vi "AlAs-GaAs superlattice-111203 a.vi"() -> ()   [LabVIEW 2011]
panel:
  in  "Number of \nGrowth Steps":i32=50
  out "step number":i32
  in  "Aluminum Flow":dbl=10.0
  in  "Ga Flow 1":dbl=5.49
  in  "As_Gas Flow":dbl=33.0
  in  "Manifold H2 Flow":dbl=700.0
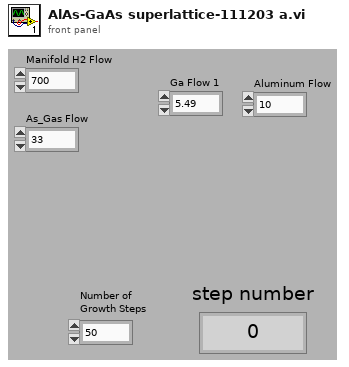
[diagram p1: front panel]
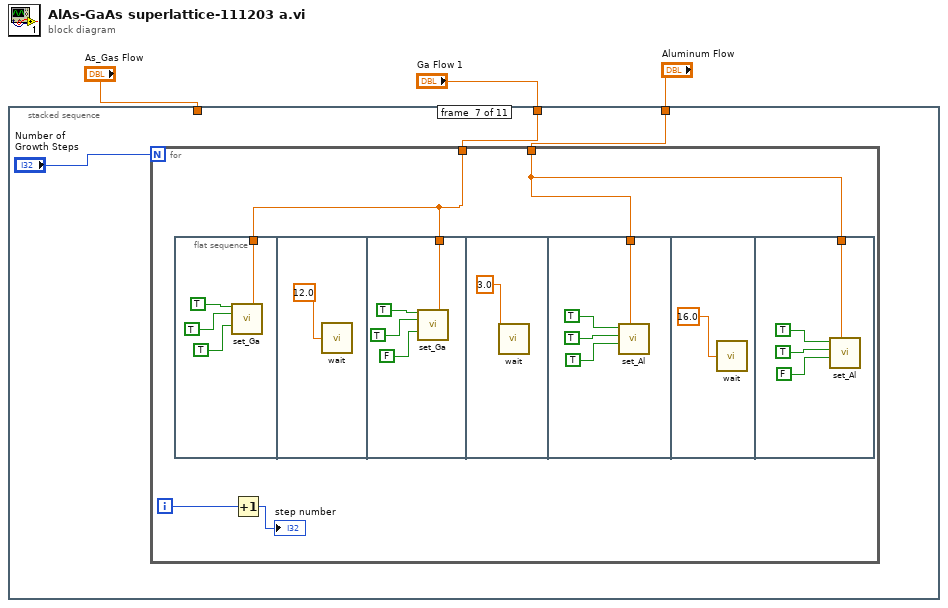
[diagram p0: block diagram]
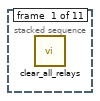
[diagram p2: hidden frame]
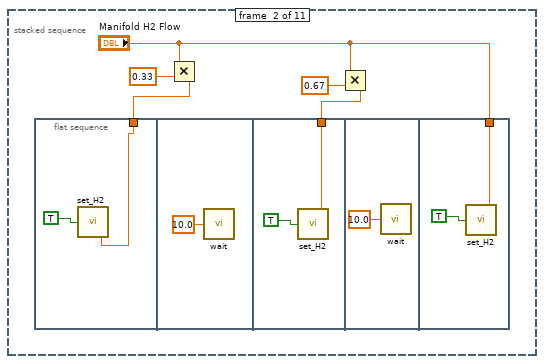
[diagram p3: hidden frame]
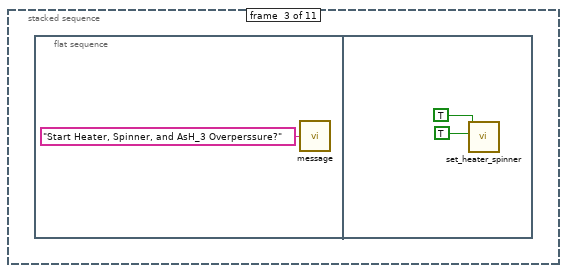
[diagram p4: hidden frame]
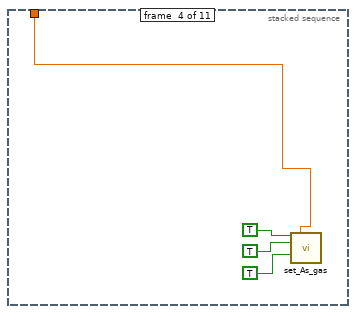
[diagram p5: hidden frame]
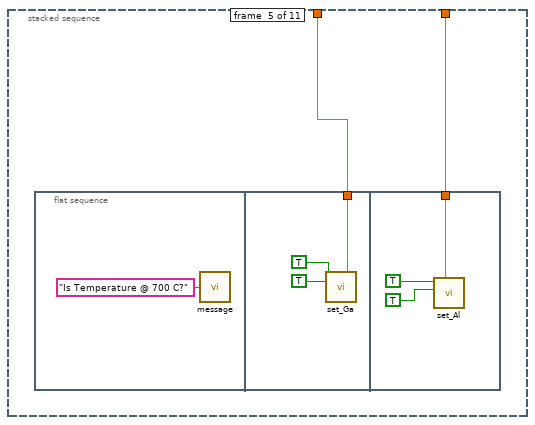
[diagram p6: hidden frame]
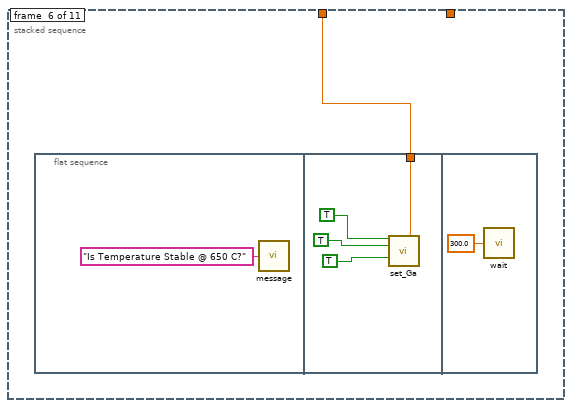
[diagram p7: hidden frame]
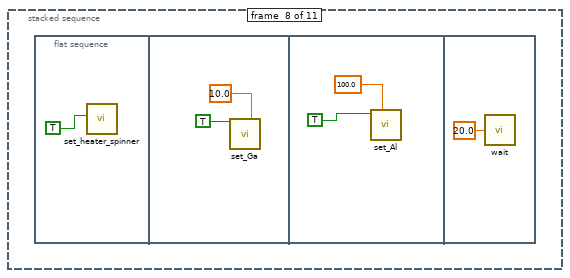
[diagram p8: hidden frame]
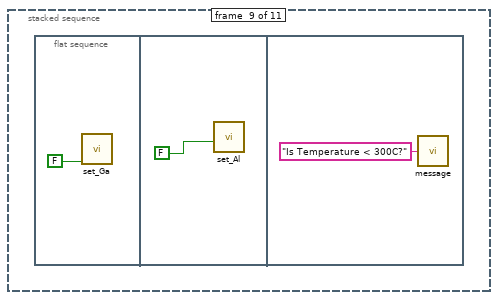
[diagram p9: hidden frame]
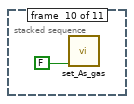
[diagram p10: hidden frame]
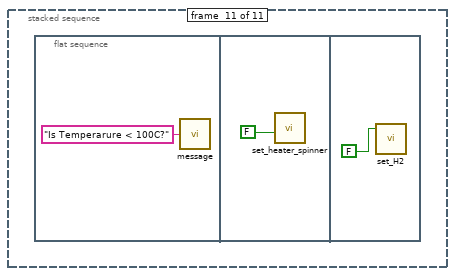
[diagram p11: hidden frame]
diagram:
  n1 = stacked-sequence {
    tunnel: "Ga Flow 1" -> [_ _ _ _ w25 w33 w41 _ _ _ _]
    tunnel: "As_Gas Flow" -> [_ _ _ w20 _ _ _ _ _ _ _]
    tunnel: "Aluminum Flow" -> [_ _ _ _ w24 _ w40 _ _ _ _]
    frame #0 {
      n2 = call "clear_all_relays.vi"() -> ()  [unwired: 2 out]
    }
    frame #1 {
      n3 = flat-sequence {
        tunnel: w8 -> [w9]
        tunnel: w6 -> [w12]
        tunnel: "Manifold H2 Flow" -> [w15]
        frame #0 {
          n4 = call "set_H2.vi"("Manifold H2 Flow"=w9, "H2 Active"=TRUE) -> ()  [unwired: 2 in, 2 out]
        }
        frame #1 {
          n5 = call "wait.vi"("Wait (s)"=10.0) -> ()
        }
        frame #2 {
          n6 = call "set_H2.vi"("Manifold H2 Flow"=w12, "H2 Active"=TRUE) -> ()  [unwired: 2 in, 2 out]
        }
        frame #3 {
          n7 = call "wait.vi"("Wait (s)"=10.0) -> ()
        }
        frame #4 {
          n8 = call "set_H2.vi"("Manifold H2 Flow"=w15, "H2 Active"=TRUE) -> ()  [unwired: 2 in, 2 out]
        }
      }
      n9 = Multiply(x="Manifold H2 Flow", y=0.33) -> (x*y=w8:dbl)
      n10 = Multiply(x="Manifold H2 Flow", y=0.67) -> (x*y=w6:dbl)
    }
    frame #2 {
      n11 = flat-sequence {
        frame #0 {
          n12 = call "message.vi"("message"="Start Heater, Spinner, and AsH_3 Overperssure?") -> ()
        }
        frame #1 {
          n13 = call "set_heater_spinner.vi"("Spinner"=TRUE, "Heater"=TRUE) -> ()  [unwired: 1 in, 7 out]
        }
      }
    }
    frame #3 {
      n14 = call "set_As_gas.vi"("As_Gas Active"=TRUE, "As_Gas Flow"=w20, "As_Gas In"=TRUE, "As_Gas Run"=TRUE) -> ()  [unwired: 2 in, 10 out]
    }
    frame #4 {
      n15 = flat-sequence {
        tunnel: w25 -> [w27]
        tunnel: w24 -> [w30]
        frame #0 {
          n16 = call "message.vi"("message"="Is Temperature @ 700 C?") -> ()
        }
        frame #1 {
          n17 = call "set_Ga.vi"("Ga Active"=TRUE, "Ga Flow 1"=w27, "Ga Bubbler"=TRUE) -> ()  [unwired: 5 in, 8 out]
        }
        frame #2 {
          n18 = call "set_Al.vi"("Aluminum Flow"=w30, "Al Bubbler"=TRUE ("Ga Bubbler"), "Al Active"=TRUE ("Ga Active")) -> ()  [unwired: 2 in, 5 out]
        }
      }
    }
    frame #5 {
      n19 = flat-sequence {
        tunnel: w33 -> [w35]
        frame #0 {
          n20 = call "message.vi"("message"="Is Temperature Stable @ 650 C?") -> ()
        }
        frame #1 {
          n21 = call "set_Ga.vi"("Ga Active"=TRUE ("P_Gas Active"), "Ga Flow 1"=w35, "Ga Bubbler"=TRUE ("P_Gas In"), "Ga Run"=TRUE ("P_Gas Run")) -> ()  [unwired: 4 in, 8 out]
        }
        frame #2 {
          n22 = call "wait.vi"("Wait (s)"=300.0) -> ()
        }
      }
    }
    frame #6 {
      n23 = for {
        N: "Number of \nGrowth Steps" -> [_]
        tunnel: w41 -> [w44]
        tunnel: w40 -> [w43]
        i -> [w45]
        n24 = flat-sequence {
          tunnel: w44 -> [w47]
          tunnel: w44 -> [w52]
          tunnel: w43 -> [w57]
          tunnel: w43 -> [w62]
          frame #0 {
            n25 = call "set_Ga.vi"("Ga Active"=TRUE ("P_Gas Active"), "Ga Flow 1"=w47, "Ga Bubbler"=TRUE ("P_Gas In"), "Ga Run"=TRUE ("P_Gas Run")) -> ()  [unwired: 4 in, 8 out]
          }
          frame #1 {
            n26 = call "wait.vi"("Wait (s)"=12.0) -> ()
          }
          frame #2 {
            n27 = call "set_Ga.vi"("Ga Active"=TRUE ("P_Gas Active"), "Ga Flow 1"=w52, "Ga Bubbler"=TRUE ("P_Gas In"), "Ga Run"=FALSE ("P_Gas Run")) -> ()  [unwired: 4 in, 8 out]
          }
          frame #3 {
            n28 = call "wait.vi"("Wait (s)"=3.0) -> ()
          }
          frame #4 {
            n29 = call "set_Al.vi"("Aluminum Flow"=w57, "Al Run"=TRUE ("P_Gas Run"), "Al Bubbler"=TRUE ("P_Gas In"), "Al Active"=TRUE ("P_Gas Active")) -> ()  [unwired: 1 in, 5 out]
          }
          frame #5 {
            n30 = call "wait.vi"("Wait (s)"=16.0) -> ()
          }
          frame #6 {
            n31 = call "set_Al.vi"("Aluminum Flow"=w62, "Al Run"=FALSE ("P_Gas Run"), "Al Bubbler"=TRUE ("P_Gas In"), "Al Active"=TRUE ("P_Gas Active")) -> ()  [unwired: 1 in, 5 out]
          }
        }
        n32 = Increment(x=w45) -> (x+1=→"step number":i32)
      }
    }
    frame #7 {
      n33 = flat-sequence {
        frame #0 {
          n34 = call "set_heater_spinner.vi"("Spinner"=TRUE ("Ga Active")) -> ()  [unwired: 2 in, 7 out]
        }
        frame #1 {
          n35 = call "set_Ga.vi"("Ga Active"=TRUE, "Ga Flow 1"=10.0) -> ()  [unwired: 6 in, 8 out]
        }
        frame #2 {
          n36 = call "set_Al.vi"("Aluminum Flow"=100.0, "Al Active"=TRUE ("Ga Active")) -> ()  [unwired: 3 in, 5 out]
        }
        frame #3 {
          n37 = call "wait.vi"("Wait (s)"=20.0) -> ()
        }
      }
    }
    frame #8 {
      n38 = flat-sequence {
        frame #0 {
          n39 = call "set_Ga.vi"("Ga Remote"=FALSE) -> ()  [unwired: 7 in, 8 out]
        }
        frame #1 {
          n40 = call "set_Al.vi"("Al Run"=FALSE ("Ga Remote")) -> ()  [unwired: 4 in, 5 out]
        }
        frame #2 {
          n41 = call "message.vi"("message"="Is Temperature < 300C?") -> ()
        }
      }
    }
    frame #9 {
      n42 = call "set_As_gas.vi"("As_Gas Remote"=FALSE) -> ()  [unwired: 5 in, 10 out]
    }
    frame #10 {
      n43 = flat-sequence {
        frame #0 {
          n44 = call "message.vi"("message"="Is Temperarure < 100C?") -> ()
        }
        frame #1 {
          n45 = call "set_heater_spinner.vi"("Heater/Spinner Remote"=FALSE) -> ()  [unwired: 2 in, 7 out]
        }
        frame #2 {
          n46 = call "set_H2.vi"("H2N2 Remote"=FALSE) -> ()  [unwired: 3 in, 2 out]
        }
      }
    }
  }
